vi "Test Boolean.vi"(7 "Name":string="Test Boolean", 10 "Succeed State":T1, 11 "Abs_Boolean.lvclass":refnum<class "Abs_Boolean.lvclass">) -> (3 "abs_Node":refnum<class "abs_Node.lvclass">)   [LabVIEW 2021, in "BT.lvlib"]
uses:
  BT.lvlib
  Support/abs_Node/abs_Node.lvclass
  LV_Abstract/Source/Abs_Types/Boolean/Abs_Boolean.lvclass
  C:/Users/Tim/Documents/GitHub/LV_Abstract/Source/Abs_Types/Type/Abs_Type.lvclass
  <vilib>/TSA/Behaviour Tree/abs_Test Boolean/Support/Succeed State.ctl
  Support/Test Boolean/Test Boolean.lvclass
  C:/Users/Tim/Documents/GitHub/LV_Behaviour_Tree/Source/Support/abs_Type Leaf/abs_Type Leaf.lvclass
  C:/Users/Tim/Documents/GitHub/LV_Behaviour_Tree/Source/Support/abs_Node/abs_Node.lvclass
  Support/abs_Type Leaf/abs_Type Leaf.lvclass/abs_Type Leaf.ctl
  LV_Abstract/Source/Abs_Types/Type/Abs_Type.lvclass/Abs_Type.ctl
  Support/abs_Type Leaf/Properties/Write Value Class.vi
  LV_Abstract/Source/Abs_Types/Type/Properties/Write Name.vi
  LV_Abstract/Source/Functions/Logic/Support/NOT/Bool/Method.vi
  LV_Abstract/Source/Functions/Logic/Support/NOT/Bool/NOT_Bool.lvclass
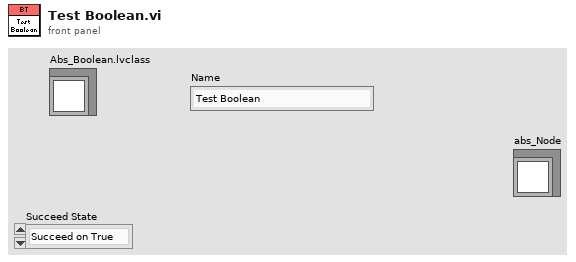
[diagram p1: front panel]
types:
  T1 = typedef "Test Boolean.lvclass/Succeed State.ctl" = enum16{"Succeed on True", "Succeed on False"}
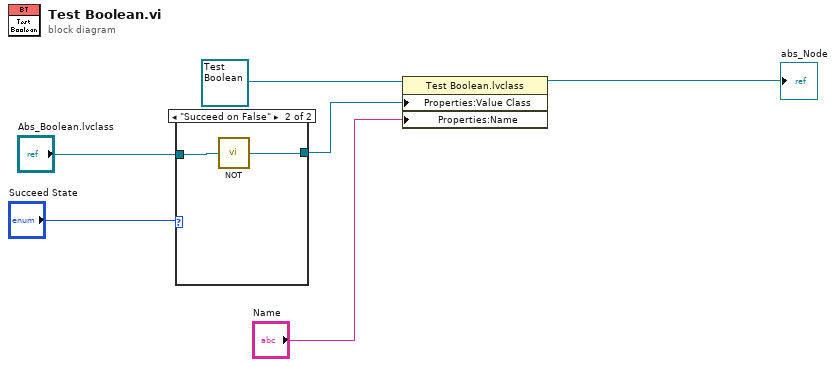
[diagram p0: block diagram]
diagram:
  n1 = case shown="\"Succeed on False\"" "Succeed State" {
    tunnel: "Abs_Boolean.lvclass" -> [w7 w9]
    tunnel: [w7 w8] -> w1
    frame "Succeed on True", Default {
    }
    frame "Succeed on False" {
      n2 = call-poly "NOT.vi"("Bool"=w9) -> ("Result"=w8:refnum<class "Abs_Boolean.lvclass">)  [unwired: 4 in]
    }
  }
  n3 = property class="Test Boolean.lvclass"(reference=refnum<class "Test Boolean.lvclass"> refnum ("BT.lvlib:Test Boolean.lvclass"), "Properties:Value Class"=w1, "Properties:Name"="Name") -> (reference out=→"abs_Node":refnum<class "Test Boolean.lvclass">)  [unwired: 1 in, 1 out]
